vi "System Status.vi"(8 "error in (no error)":errorcluster, 11 "VISA resource name":refnum<visa-resource-name>) -> (0 "error out":errorcluster, 1 "Any Error? (F)":bool, 2 "ESR? (0)":i32 format="%.0b", 3 "VISA resource name out":refnum<visa-resource-name>)   [LabVIEW 2017, in "Agilent 4194.lvlib"]
doc: "This function reads the Standard Event Register and checks it for error occurrence."
uses:
  Agilent 4194.lvlib
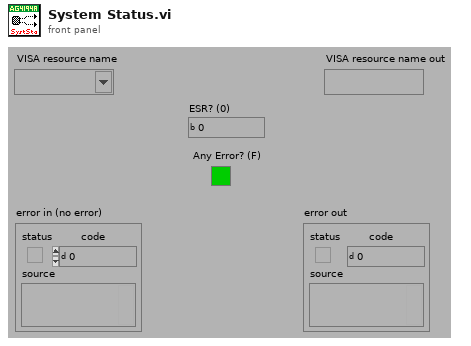
[diagram p1: front panel]
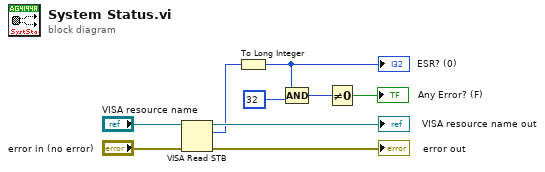
[diagram p0: block diagram]
diagram:
  n1 = VISA Read STB(8:"error in (no error)", 11:"VISA resource name") -> (0:→"error out":errorcluster, 2:w4:u16, 3:→"VISA resource name out":refnum<visa-resource-name>)
  n2 = To Long Integer(number=w4) -> (32bit integer=w3:i32)
  "ESR? (0)" <- w3
  n3 = Compound Arithmetic op=AND(w3, 32 ("y")) -> (w2:i32)
  n4 = Not Equal To 0?(x=w2) -> (x != 0?=→"Any Error? (F)":bool)
